vi "_Translate Turbo Error.vi"(1 "Error Code":string) -> (0 "Translation":string)   [LabVIEW 2012]
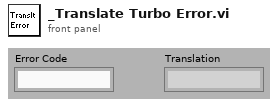
[diagram p1: front panel]
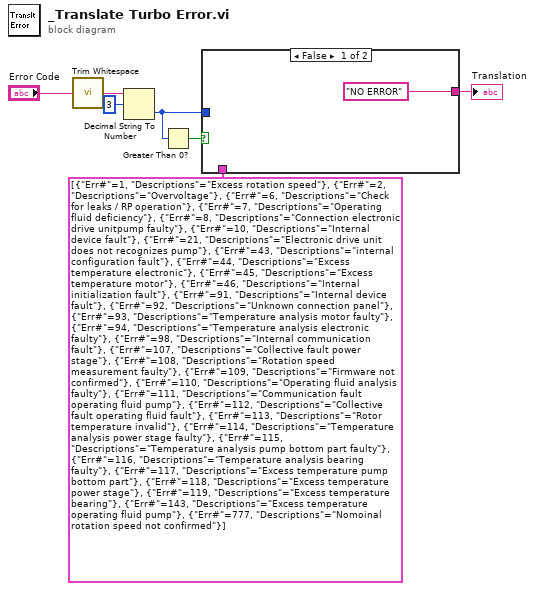
[diagram p0: block diagram]
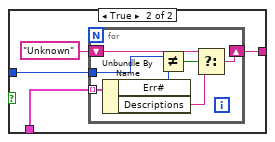
[diagram p2: hidden frame]
diagram:
  n1 = call <vilib>:"Trim Whitespace.vi"("string"="Error Code") -> ("trimmed string"=w3:string)  [unwired: 1 in]
  n2 = Decimal String To Number(string=w3, offset=3 ("offset (0)")) -> (number=w5:i32)  [unwired: 2 out]
  n3 = Greater Than 0?(x=w5) -> (x > 0?=w4:bool)
  n4 = case shown="False" w4 {
    tunnel: w5 -> [_ w12]
    tunnel: cluster{"Err#":i32, "Descriptions":string}[] [{"Err#"=1, "Descriptions"="Excess rotation speed"}, {"Err#"=2, "Descriptions"="Overvoltage"}, {"Err#"=6, "Descriptions"="Check for leaks / RP operation"}, {"Err#"=7, "Descriptions"="Operating fluid deficiency"}, {"Err#"=8, "Descriptions"="Connection electronic drive unitpump faulty"}, {"Err#"=10, "Descriptions"="Internal device fault"}, {"Err#"=21, "Descriptions"="Electronic drive unit does not recognizes pump"}, {"Err#"=43, "Descriptions"="internal configuration fault"}, {"Err#"=44, "Descriptions"="Excess temperature electronic"}, {"Err#"=45, "Descriptions"="Excess temperature motor"}, {"Err#"=46, "Descriptions"="Internal initialization fault"}, {"Err#"=91, "Descriptions"="Internal device fault"}, {"Err#"=92, "Descriptions"="Unknown connection panel"}, {"Err#"=93, "Descriptions"="Temperature analysis motor faulty"}, {"Err#"=94, "Descriptions"="Temperature analysis electronic faulty"}, {"Err#"=98, "Descriptions"="Internal communication fault"}, {"Err#"=107, "Descriptions"="Collective fault power stage"}, {"Err#"=108, "Descriptions"="Rotation speed measurement faulty"}, {"Err#"=109, "Descriptions"="Firmware not confirmed"}, {"Err#"=110, "Descriptions"="Operating fluid analysis faulty"}, {"Err#"=111, "Descriptions"="Communication fault operating fluid pump"}, {"Err#"=112, "Descriptions"="Collective fault operating fluid fault"}, {"Err#"=113, "Descriptions"="Rotor temperature invalid"}, {"Err#"=114, "Descriptions"="Temperature analysis power stage faulty"}, {"Err#"=115, "Descriptions"="Temperature analysis pump bottom part faulty"}, {"Err#"=116, "Descriptions"="Temperature analysis bearing faulty"}, {"Err#"=117, "Descriptions"="Excess temperature pump bottom part"}, {"Err#"=118, "Descriptions"="Excess temperature power stage"}, {"Err#"=119, "Descriptions"="Excess temperature bearing"}, {"Err#"=143, "Descriptions"="Excess temperature operating fluid pump"}, {"Err#"=777, "Descriptions"="Nomoinal rotation speed not confirmed"}] ("Array") -> [_ w11]
    tunnel: ["NO ERROR" w9] -> w7
    frame False {
    }
    frame True {
      n5 = for {
        tunnel: w12 -> [w19]
        tunnel: w11 -> [w18] mode=indexing
        shift-right: [w13] -> w9
        shift-left: "Unknown" -> [w15]
        n6 = Unbundle By Name(w18) -> ("Err#"=w17:i32, "Descriptions"=w14:string)
        n7 = Not Equal?(x=w19, y=w17) -> (x != y?=w16:bool)
        n8 = Select(t=w15, s=w16, f=w14) -> (s? t:f=w13:string)
      }
    }
  }
  "Translation" <- w7
